vi "FdxCmdMonGetStatusCvi.vi"(8 "error in":errorcluster, 11 "InstrumentHandle_port":u32) -> (0 "error out":errorcluster, 1 "MonStatus":T1 {"MonStatus" items=["FDX_MON_OFF", "FDX_MON_WAIT_FOR_TRIGGER", "FDX_MON_TRIGGERED", "FDX_MON_STOPPED", "FDX_MON_FULL", "FDX_MON_OVERLOAD"]}, 3 "InstrumentHandle_port":u32)   [LabVIEW 2020, in "AIM664LV.lvlib"]
doc: "This function returns the status of the selected receiver monitor port."
uses:
  AIM664LV.lvlib
  AFDX_LibraryAdmin/FdxGlobalDllPath.vi
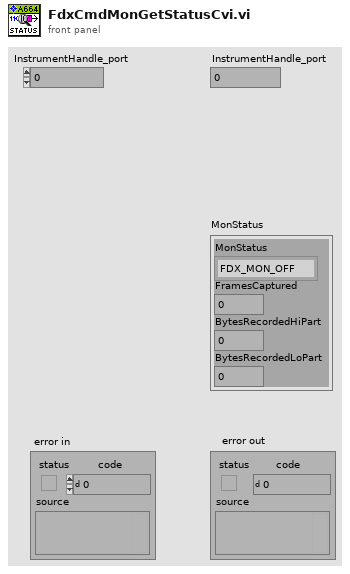
[diagram p1: front panel]
types:
  T1 = cluster{"MonStatus":u32, "FramesCaptured":u32, "BytesRecordedHiPart":u32, "BytesRecordedLoPart":u32}
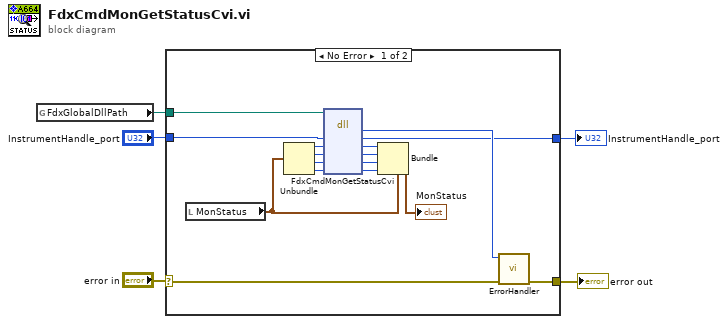
[diagram p0: block diagram]
diagram:
  n1 = global read "FdxGlobalDllPath.vi" "FdxGlobalDllPath"() -> (w3:path)
  n2 = case shown="No Error" "error in" {
    selector: "error in" -> [w20 w23]
    tunnel: [w21 w23] -> w5
    tunnel: w3 -> [w8 _]
    tunnel: "InstrumentHandle_port" -> [w7 w22]
    tunnel: [w6 w22] -> w1
    frame No Error {
      n3 = local read "MonStatus"() -> (w9:T1)
      n4 = Unbundle(w9) -> ("MonStatus"=w13:u32, "FramesCaptured"=w12:u32, "BytesRecordedHiPart"=w11:u32, "BytesRecordedLoPart"=w10:u32)
      n5 = dll-call lib="aim_fdx.19.dll" fn="FdxCmdMonGetStatusCvi"(path in=w8, "InstrumentHandle"=w7, "MonStatus"=w13, "FramesCaptured"=w12, "BytesRecordedHiPart"=w11, "BytesRecordedLoPart"=w10) -> ("status"=w19:i32, "InstrumentHandle"=w6:u32, "MonStatus"=w15:u32, "FramesCaptured"=w16:u32, "BytesRecordedHiPart"=w17:u32, "BytesRecordedLoPart"=w18:u32)  [unwired: 2 in, 2 out]
      n6 = Bundle(cluster=w9, "MonStatus"=w15, "FramesCaptured"=w16, "BytesRecordedHiPart"=w17, "BytesRecordedLoPart"=w18) -> (→"MonStatus":T1)
      n7 = call "ErrorHandler.vi"("error in"=w20, "AIM Error"=w19) -> ("error out"=w21:errorcluster)  [unwired: 9 in]
    }
    frame Error {
    }
  }
  "error out" <- w5
  "InstrumentHandle_port" <- w1
